vi "BERT Ch Restart subVI.vi"(11 "error in (no error)":errorcluster) -> (3 "error out":errorcluster)   [LabVIEW 2010]
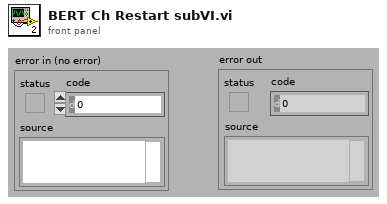
[diagram p1: front panel]
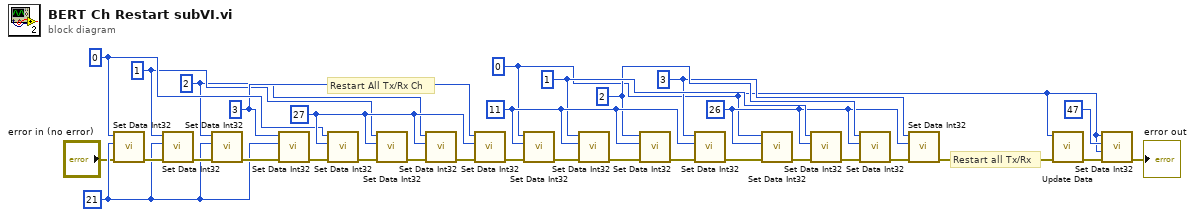
[diagram p0: block diagram]
diagram:
  w3 = 3
  w1 = 2
  w4 = 0
  w2 = 1
  w9 = 26
  w10 = 3
  w11 = 2
  w12 = 1
  w7 = 0
  w20 = 11
  w24 = 27
  w25 = 21
  # "Restart all Tx/Rx"
  # "Restart All Tx/Rx Ch"
  n1 = call <instrlib>:"Set Data Int32.vi"("error in (no error)"="error in (no error)", "func"=w25, "chan"=w4) -> ("error out"=w32:errorcluster)  [unwired: 7 in, 1 out]
  n2 = call <instrlib>:"Set Data Int32.vi"("error in (no error)"=w32, "func"=w25, "chan"=w2) -> ("error out"=w31:errorcluster)  [unwired: 7 in, 1 out]
  n3 = call <instrlib>:"Set Data Int32.vi"("error in (no error)"=w31, "func"=w25, "chan"=w1) -> ("error out"=w30:errorcluster)  [unwired: 7 in, 1 out]
  n4 = call <instrlib>:"Set Data Int32.vi"("error in (no error)"=w30, "func"=w25, "chan"=w3) -> ("error out"=w29:errorcluster)  [unwired: 7 in, 1 out]
  n5 = call <instrlib>:"Set Data Int32.vi"("error in (no error)"=w29, "func"=w24, "chan"=w4) -> ("error out"=w28:errorcluster)  [unwired: 7 in, 1 out]
  n6 = call <instrlib>:"Set Data Int32.vi"("error in (no error)"=w28, "func"=w24, "chan"=w2) -> ("error out"=w27:errorcluster)  [unwired: 7 in, 1 out]
  n7 = call <instrlib>:"Set Data Int32.vi"("error in (no error)"=w27, "func"=w24, "chan"=w1) -> ("error out"=w26:errorcluster)  [unwired: 7 in, 1 out]
  n8 = call <instrlib>:"Set Data Int32.vi"("error in (no error)"=w26, "func"=w24, "chan"=w3) -> ("error out"=w8:errorcluster)  [unwired: 7 in, 1 out]
  n9 = call <instrlib>:"Set Data Int32.vi"("error in (no error)"=w8, "func"=w20, "chan"=w7) -> ("error out"=w23:errorcluster)  [unwired: 7 in, 1 out]
  n10 = call <instrlib>:"Set Data Int32.vi"("error in (no error)"=w23, "func"=w20, "chan"=w12) -> ("error out"=w22:errorcluster)  [unwired: 7 in, 1 out]
  n11 = call <instrlib>:"Set Data Int32.vi"("error in (no error)"=w22, "func"=w20, "chan"=w11) -> ("error out"=w21:errorcluster)  [unwired: 7 in, 1 out]
  n12 = call <instrlib>:"Set Data Int32.vi"("error in (no error)"=w21, "func"=w20, "chan"=w10) -> ("error out"=w17:errorcluster)  [unwired: 7 in, 1 out]
  n13 = call <instrlib>:"Set Data Int32.vi"("error in (no error)"=w17, "func"=w9, "chan"=w7) -> ("error out"=w16:errorcluster)  [unwired: 7 in, 1 out]
  n14 = call <instrlib>:"Set Data Int32.vi"("error in (no error)"=w16, "func"=w9, "chan"=w12) -> ("error out"=w15:errorcluster)  [unwired: 7 in, 1 out]
  n15 = call <instrlib>:"Set Data Int32.vi"("error in (no error)"=w15, "func"=w9, "chan"=w11) -> ("error out"=w14:errorcluster)  [unwired: 7 in, 1 out]
  n16 = call <instrlib>:"Set Data Int32.vi"("error in (no error)"=w14, "func"=w9, "chan"=w10) -> ("error out"=w13:errorcluster)  [unwired: 7 in, 1 out]
  n17 = call <instrlib>:"Update Data.vi"("error in (no error)"=w13, "type"=w7) -> ("error out"=w19:errorcluster)  [unwired: 8 in, 1 out]
  n18 = call <instrlib>:"Set Data Int32.vi"("error in (no error)"=w19, "value"=w7, "func"=47, "chan"=w7) -> ("error out"=→"error out":errorcluster)  [unwired: 6 in, 1 out]
